vi "ByPassCom.vi"(8 "error in (no error)":errorcluster, 10 "Param":string, 11 "COMM in":refnum<class "COMM.lvclass">) -> (0 "error out":errorcluster, 2 "Resp":string, 3 "COMM out":refnum<class "COMM.lvclass">)   [LabVIEW 2018, in "COMM.lvclass"]
uses:
  COMM.lvclass
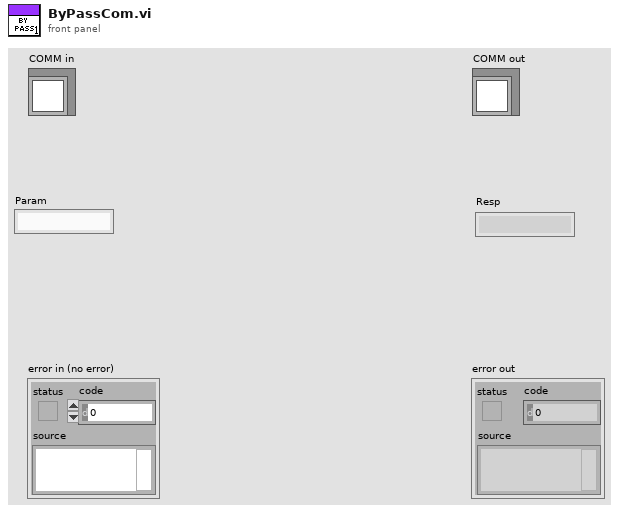
[diagram p1: front panel]
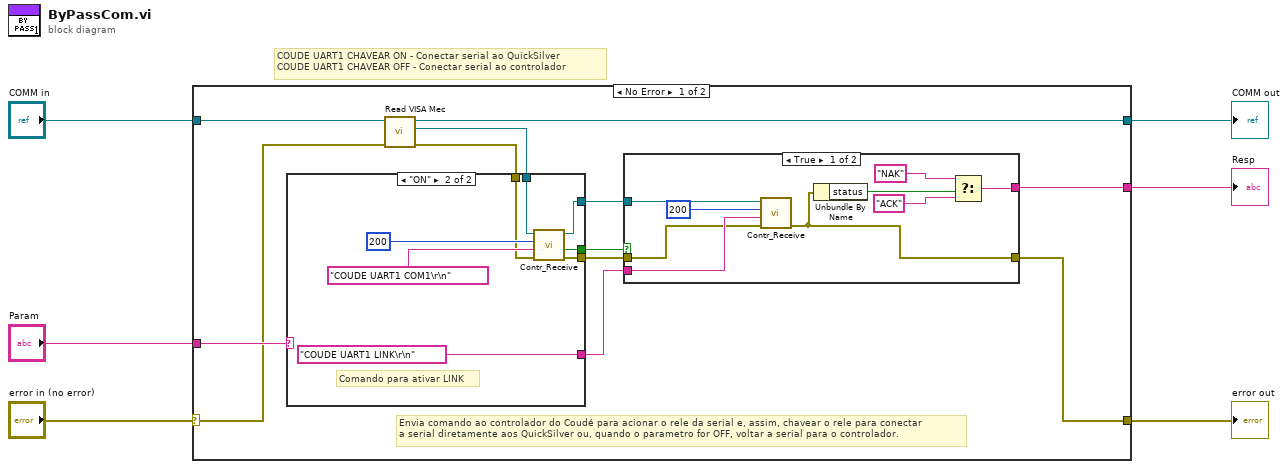
[diagram p0: block diagram]
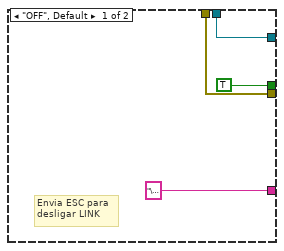
[diagram p2: hidden frame]
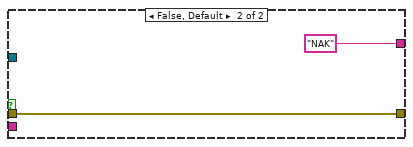
[diagram p3: hidden frame]
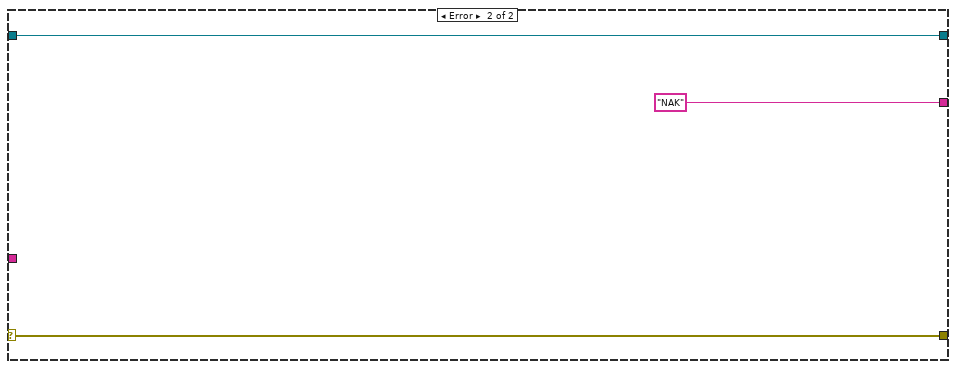
[diagram p4: hidden frame]
diagram:
  # "COUDE UART1 CHAVEAR ON - Conectar serial ao QuickSilver\nCOUDE UART1 CHAVEAR OFF - Conectar serial ao controlador"
  n1 = case shown="No Error" "error in (no error)" {
    selector: "error in (no error)" -> [w9 w43]
    tunnel: "COMM in" -> [w11 w44]
    tunnel: [w10 w44] -> w4
    tunnel: [w18 w43] -> w2
    tunnel: "Param" -> [w16 _]
    tunnel: [w17 "NAK"] -> w3
    frame No Error {
      # "Envia comando ao controlador do Coudé para acionar o rele da serial e, assim, chavear o rele para conectar \na serial diretamente aos QuickSilver ou, quando o parametro for OFF, voltar a serial para o controlador."
      n2 = call-dynamic "Read VISA Mec.vi"("error in (no error)"=w9, "Controlador in"=w11) -> ("error out"=w7:errorcluster, "VISA Mec"=w8:refnum<visa-resource-name>, "Controlador out"=w10:refnum<class "COMM.lvclass">)  [unwired: 7 in]
      n3 = case shown="\"ON\"" w16 {
        tunnel: ["\u001b" ("Command to SIFS") "COUDE UART1 LINK\r\n" ("Command to SIFS")] -> w15
        tunnel: [w21 w23] -> w13
        tunnel: [w19 w25] -> w14
        tunnel: w8 -> [w21 w29]
        tunnel: [TRUE ("cmd sent") w24] -> w12
        tunnel: w7 -> [w19 w26]
        frame "OFF", Default {
          # "Envia ESC para \ndesligar LINK"
        }
        frame "ON" {
          # "Comando para ativar LINK"
          n4 = call "Contr_Receive.vi"("error in"=w26, "Command to SIFS"="COUDE UART1 COM1\r\n", "wait after tx"=u32 200 ("milliseconds to wait"), "VISA resource name"=w29) -> ("error out"=w25:errorcluster, "cmd sent"=w24:bool, "VISA resource name out"=w23:refnum<visa-resource-name>)  [unwired: 1 out]
        }
      }
      n5 = case shown="True" w12 {
        tunnel: [w31 w41] -> w18
        tunnel: w14 -> [w32 w41]
        tunnel: w13 -> [w35 _]
        tunnel: [w39 "NAK"] -> w17
        tunnel: w15 -> [w33 _]
        frame True {
          n6 = call "Contr_Receive.vi"("error in"=w32, "Command to SIFS"=w33, "wait after tx"=u32 200 ("milliseconds to wait"), "VISA resource name"=w35) -> ("error out"=w31:errorcluster)  [unwired: 3 out]
          n7 = Unbundle By Name(w31) -> ("status"=w36:bool)
          n8 = Select(t="NAK", s=w36, f="ACK") -> (s? t:f=w39:string)
        }
        frame False, Default {
        }
      }
    }
    frame Error {
    }
  }
  "error out" <- w2
  "COMM out" <- w4
  "Resp" <- w3
